vi "Helper Loop Create.vi"(10 "Helper Loop":refnum<class "Helper Loop.lvclass">, 11 "Dev Actor in":refnum<class "Dev Actor.lvclass">) -> (3 "Dev Actor out":refnum<class "Dev Actor.lvclass">)   [LabVIEW 2021, in "Dev Actor.lvlib" / "Dev Actor.lvclass"]
uses:
  Dev Actor.lvclass
  Helper Loop/Helper Loop/Helper Loop.lvclass
  Dev Actor.lvclass/Dev Actor.ctl
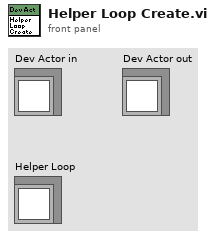
[diagram p1: front panel]
types:
  T1 = typedef "Dev Actor Refs.ctl" = cluster{"Pop Up":refnum<vi>, "String Indicator":refnum<vi>}
  T2 = typedef "Dev Actor Events.ctl" = cluster{"Teardown":refnum<user-event>, "String Indicator":refnum<user-event>}
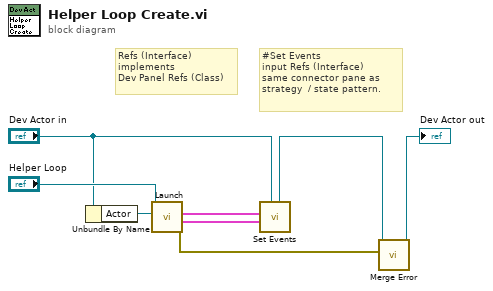
[diagram p0: block diagram]
diagram:
  # "Refs (Interface)\nimplements\nDev Panel Refs (Class)"
  # "#Set Events\ninput Refs (Interface)\nsame connector pane as strategy  / state pattern."
  n1 = Unbundle By Name("Dev Actor in") -> ("Actor"=w6:refnum<class "Actor.lvclass">)
  n2 = call "Launch.vi"("Actor"=w6, "Helper Loop in"="Helper Loop") -> ("error out"=w8:errorcluster, "Dev Actor Refs"=w1:T1, "Dev Actor Events"=w2:T2)  [unwired: 7 in]
  n3 = call "Set Events.vi"("Dev Actor in"="Dev Actor in", "Dev Actor Refs"=w1, "Dev Actor Events"=w2) -> ("Dev Actor out"=w3:refnum<class "Dev Actor.lvclass">)  [unwired: 8 in]
  n4 = call-dynamic "Merge Error.vi"("Error"=w8, "Dev Actor in"=w3) -> ("Dev Actor out"=→"Dev Actor out":refnum<class "Dev Actor.lvclass">)  [unwired: 9 in]
